vi "TurretChooseAngle.vi"() -> ()   [LabVIEW 2019]
panel:
  in  "Goal Angle (deg) 2":dbl format="%#_13g"
  in  "Deadzone Min(deg)":dbl=10.0 format="%#_13g"
  in  "Deadzone Max(deg)":dbl=10.0 format="%#_13g"
  in  "Zero Wheels":bool
  in  "Goal Angle (deg)":dbl format="%#_13g"
  in  "Current Angle (deg)":dbl format="%#_13g"
  out "Invert Speed  Motor (?)":bool
  out "Angular Distance (deg)":dbl format="%_4g"
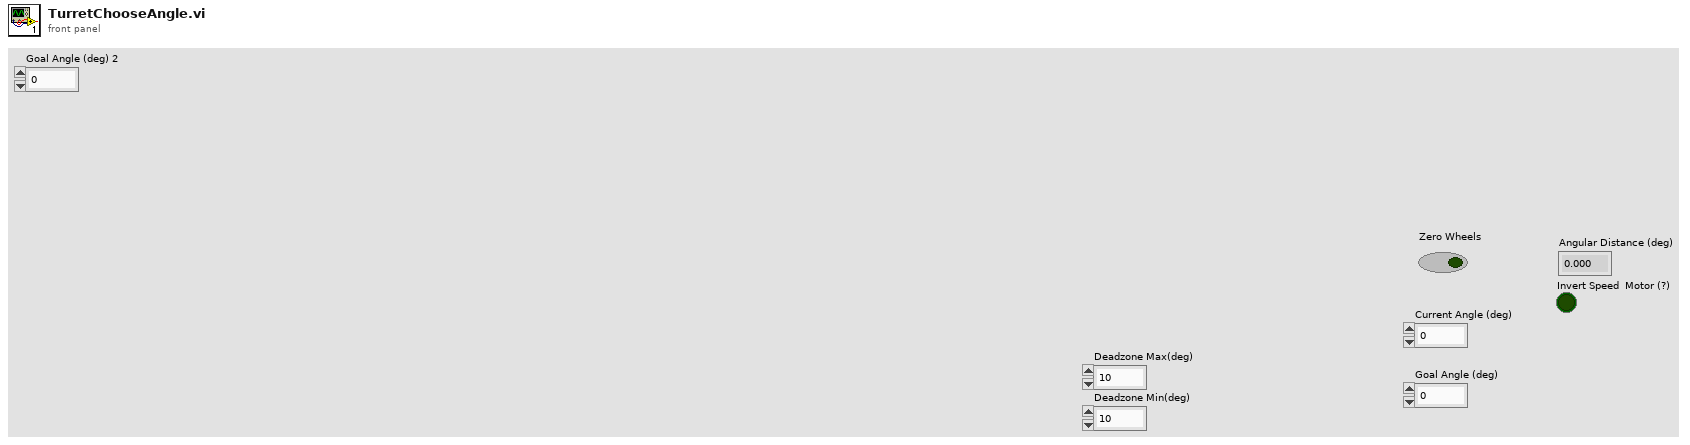
[diagram p1: front panel]
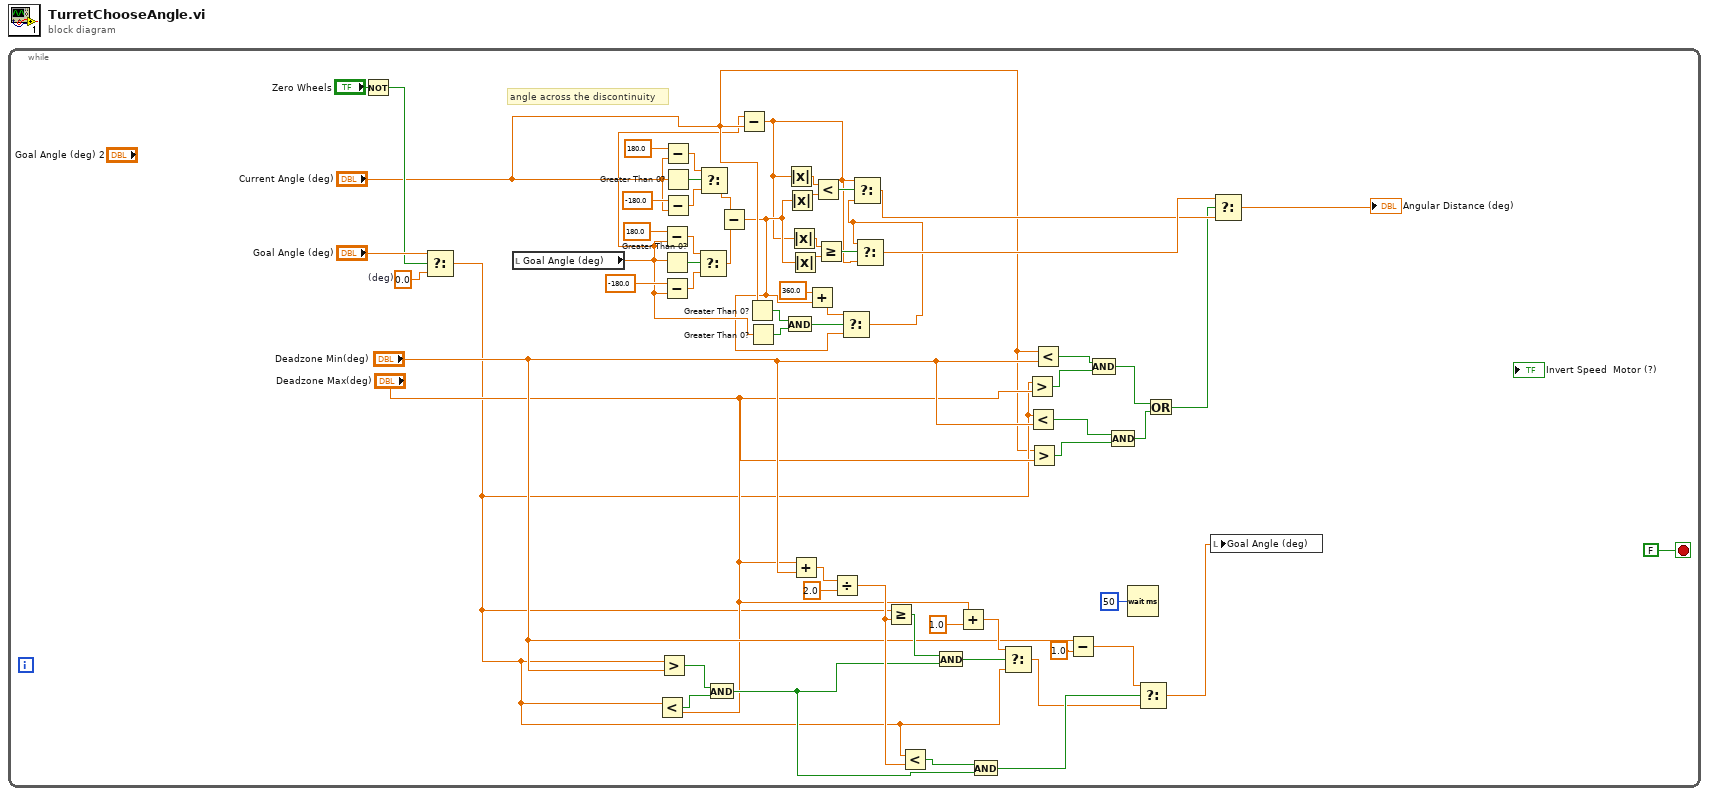
[diagram p0: block diagram]
diagram:
  n1 = while {
    stop <- FALSE stop-if-true
    w50 = 0.0  # (deg)
    # "angle across the discontinuity"
    n2 = Not(x="Zero Wheels") -> (.not. x?=w51:bool)
    n3 = Select(t="Goal Angle (deg)", s=w51, f=w50) -> (s? t:f=w11:dbl)
    n4 = local read "Goal Angle (deg)"() -> (w9:dbl)
    n5 = Less?(x=w11, y="Deadzone Max(deg)") -> (x < y?=w27:bool)
    n6 = Greater?(x=w11, y="Deadzone Min(deg)") -> (0:w26:bool)
    n7 = Subtract(x=180.0, y=w9) -> (x-y=w56:dbl)
    n8 = Greater Than 0?(x=w9) -> (x > 0?=w58:bool)
    n9 = Subtract(x=-180.0, y=w9) -> (x-y=w54:dbl)
    n10 = Subtract(x=180.0, y="Current Angle (deg)") -> (x-y=w47:dbl)
    n11 = Greater Than 0?(x="Current Angle (deg)") -> (x > 0?=w61:bool)
    n12 = Subtract(x=-180.0, y="Current Angle (deg)") -> (x-y=w46:dbl)
    n13 = Select(t=w56, s=w58, f=w54) -> (s? t:f=w45:dbl)
    n14 = Select(t=w47, s=w61, f=w46) -> (s? t:f=w44:dbl)
    n15 = And(x=w26, y=w27) -> (x .and. y?=w19:bool)
    n16 = Subtract(x=w44, y=w45) -> (x-y=w3:dbl)
    n17 = Subtract(x=w9, y="Current Angle (deg)") -> (x-y=w2:dbl)
    n18 = Greater Than 0?(x="Current Angle (deg)") -> (x > 0?=w7:bool)
    n19 = Greater Than 0?(x=w9) -> (x > 0?=w8:bool)
    n20 = And(x=w7, y=w8) -> (x .and. y?=w6:bool)
    n21 = Absolute Value(x=w2) -> (abs(x)=w62:dbl)
    n22 = Absolute Value(x=w3) -> (abs(x)=w63:dbl)
    n23 = Absolute Value(x=w2) -> (abs(x)=w36:dbl)
    n24 = Absolute Value(x=w3) -> (abs(x)=w37:dbl)
    n25 = Add(x="Deadzone Max(deg)", y="Deadzone Min(deg)") -> (x+y=w29:dbl)
    n26 = Add(x=360.0, y=w3) -> (x+y=w4:dbl)
    n27 = Less?(x=w62, y=w63) -> (x < y?=w38:bool)
    n28 = Greater Or Equal?(x=w36, y=w37) -> (x >= y?=w35:bool)
    n29 = Divide(x=w29, y=2.0) -> (x/y=w21:dbl)
    n30 = Select(t=w4, s=w6, f=w3) -> (s? t:f=w1:dbl)
    n31 = Select(t=w2, s=w38, f=w1) -> (s? t:f=w33:dbl)
    n32 = Select(t=w1, s=w35, f=w2) -> (s? t:f=w34:dbl)
    n33 = Greater Or Equal?(x=w11, y=w21) -> (x >= y?=w25:bool)
    n34 = Less?(x=w11, y=w21) -> (x < y?=w20:bool)
    n35 = And(x=w25, y=w19) -> (x .and. y?=w24:bool)
    n36 = Add(x="Deadzone Max(deg)", y=1.0) -> (x+y=w22:dbl)
    n37 = And(x=w20, y=w19) -> (x .and. y?=w18:bool)
    n38 = Select(t=w22, s=w24, f=w11) -> (s? t:f=w15:dbl)
    n39 = Greater?(x=w11, y="Deadzone Max(deg)") -> (0:w43:bool)
    n40 = Less?(x=w11, y="Deadzone Min(deg)") -> (x < y?=w40:bool)
    n41 = Greater?(x="Current Angle (deg)", y="Deadzone Max(deg)") -> (0:w41:bool)
    n42 = Less?(x="Current Angle (deg)", y="Deadzone Min(deg)") -> (x < y?=w42:bool)
    n43 = Subtract(x="Deadzone Min(deg)", y=1.0) -> (x-y=w16:dbl)
    n44 = Compound Arithmetic op=AND(w42, w43) -> (w31:bool)
    n45 = Compound Arithmetic op=AND(w40, w41) -> (w32:bool)
    n46 = Wait (ms)(milliseconds to wait=u32 50) -> ()  [unwired: 1 out]
    n47 = Select(t=w16, s=w18, f=w15) -> (s? t:f=w14:dbl)
    n48 = Or(x=w31, y=w32) -> (x .or. y?=w30:bool)
    n49 = local write "Goal Angle (deg)"(w14) -> ()
    n50 = Select(t=w34, s=w30, f=w33) -> (s? t:f=→"Angular Distance (deg)":dbl)
  }
